vi "test.vi"() -> ()   [LabVIEW 2016]
panel:
  out "date/time string":string
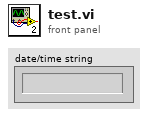
[diagram p1: front panel]
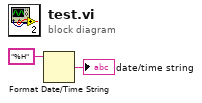
[diagram p0: block diagram]
diagram:
  n1 = Format Date/Time String(time format string (%c)="%H") -> (date/time string=→"date/time string":string)  [unwired: 2 in]
